vi "rethinkdb_tcp_parse_error.vi"(8 "error in (no error)":errorcluster, 11 "message":string) -> (0 "error out":errorcluster, 1 "is error?":bool)   [LabVIEW 2017]
uses:
  <vilib>/Utility/error.llb/Error Cluster From Error Code.vi
  <vilib>/ErrorRing/Error Ring.xnode
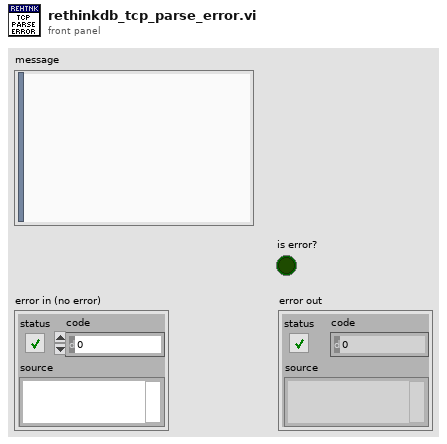
[diagram p1: front panel]
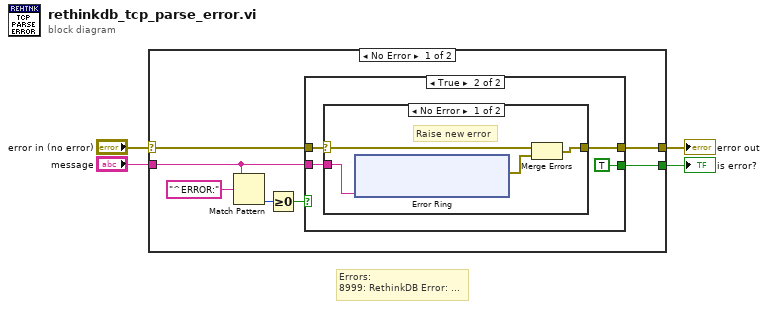
[diagram p0: block diagram]
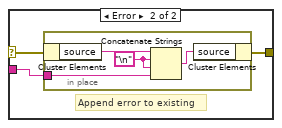
[diagram p3: hidden frame]
diagram:
  # "Errors:\n8999: RethinkDB Error: ..."
  n1 = case shown="No Error" "error in (no error)" {
    selector: "error in (no error)" -> [w11 w35]
    tunnel: [w10 w35] -> w3
    tunnel: [w9 _] -> w2
    tunnel: "message" -> [w6 _]
    frame No Error {
      n2 = Match Pattern(string=w6, regular expression="^ERROR:") -> (offset past match=w7:i32)  [unwired: 1 in, 3 out]
      n3 = Greater Or Equal To 0?(x=w7) -> (x >= 0?=w5:bool)
      n4 = case shown="True" w5 {
        tunnel: w11 -> [w12 w16]
        tunnel: w6 -> [_ w14]
        tunnel: [w12 w15] -> w10
        tunnel: [_ TRUE] -> w9
        frame False {
        }
        frame True {
          n5 = case shown="No Error" w16 {
            selector: w16 -> [w20 w30]
            tunnel: [w19 w29] -> w15
            tunnel: w14 -> [w17 w28]
            frame No Error {
              # "Raise new error"
              n6 = xnode "Error Ring"("parameter 0"=w17) -> ("error out"=w18:errorcluster)
              n7 = Merge Errors(w20, w18) -> (w19:errorcluster)
            }
            frame Error {
              # "Append error to existing"
              n8 = in-place {
                in-place-border: w28 -> [w32]
                w31 = "\n"
                n9 = in-place-cluster #1(w30) -> ("source"=w34:string)
                n10 = Concatenate Strings(w34, w31, w31, w32) -> (w33:string)
                n11 = in-place-cluster #1("source"=w33) -> (w29:errorcluster)
              }
            }
          }
        }
      }
    }
    frame Error {
    }
  }
  "error out" <- w3
  "is error?" <- w2
